vi "Digitizer Strain Configure Full Bridge Poisson Bend.vi"(0 "instrument handle":refnum<k15>, 1 "Range":dbl, 2 "Coupling (DC)":i32(ring) items=["DC", "AC"], 3 "SampCount":i32 format="%.0g", 5 "GaugeFactor":dbl, 7 "PoissonRatio":dbl, 9 "ExcitationVoltage":dbl, 10 "ChannelList":string, 11 "error in (no error)":errorcluster {"code" format="%.0x"}, 12 "InputType (Differential)":i32(ring) items=["Differential", "Sended"], 13 "Mode (Time)":i32(ring) items=["Time", "Frequency"], 14 "SampRate":dbl) -> (4 "instrument handle out":refnum<k15>, 15 "error out":errorcluster {"code" format="%.0x"})   [LabVIEW 2020, in "Keysight DAQ970.lvlib"]
doc: "Configures the channels for full bending poisson bridge strain gauge module digitizing, but they do not initiate the digitizing."
uses:
  Keysight DAQ970.lvlib
  KtDAQ970.dll
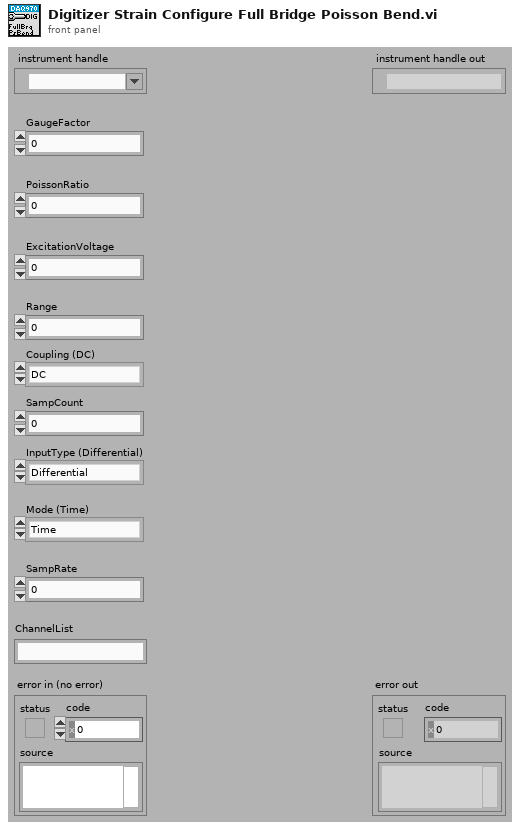
[diagram p1: front panel]
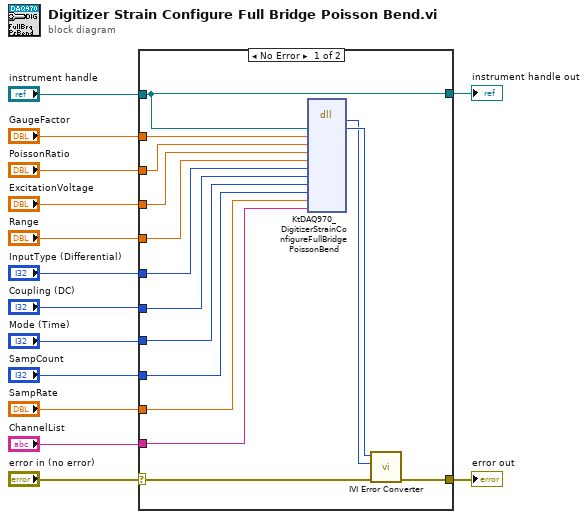
[diagram p0: block diagram]
diagram:
  n1 = case shown="No Error" "error in (no error)" {
    selector: "error in (no error)" -> [w27 w31]
    tunnel: [w26 w31] -> w14
    tunnel: "instrument handle" -> [w15 w30]
    tunnel: "GaugeFactor" -> [w25 _]
    tunnel: "PoissonRatio" -> [w24 _]
    tunnel: "ExcitationVoltage" -> [w23 _]
    tunnel: "Range" -> [w22 _]
    tunnel: "InputType (Differential)" -> [w21 _]
    tunnel: "Coupling (DC)" -> [w20 _]
    tunnel: "Mode (Time)" -> [w19 _]
    tunnel: "SampCount" -> [w18 _]
    tunnel: "SampRate" -> [w17 _]
    tunnel: "ChannelList" -> [w16 _]
    tunnel: [w15 w30] -> w1
    frame No Error {
      n2 = dll-call lib="KtDAQ970**.dll" fn="KtDAQ970_DigitizerStrainConfigureFullBridgePoissonBend"("Vi"=w15, "GaugeFactor"=w25, "PoissonRatio"=w24, "ExcitationVoltage"=w23, "Range"=w22, "InputType"=w21, "Coupling"=w20, "Mode"=w19, "SampCount"=w18, "SampRate"=w17, "ChannelList"=w16) -> (w28:i32, "Vi"=w29:u32)  [unwired: 13 in, 2 out]
      n3 = call "IVI Error Converter.vi"("error in (no error)"=w27, "IVI error code (0)"=w28, "instrument handle"=w29) -> ("error out"=w26:errorcluster)  [unwired: 7 in, 1 out]
    }
    frame Error {
    }
  }
  "error out" <- w14
  "instrument handle out" <- w1
